vi "PixelFlyTEMP.vi"() -> ()   [LabVIEW 2012]
uses:
  <vilib>/Platform/TimedLoop/XDataNode/timing_clust.ctl
  <vilib>/Platform/TimedLoop/XDataNode/nitl_modes.ctl
  <vilib>/Platform/TimedLoop/XDataNode/wakeup.ctl
  <vilib>/platform/TimedLoop/XDataNode/XDataNode.xnode
  <vilib>/Platform/TimedLoop/XDataNode/XDNodeRunTimeDep.lvlib
panel:
  in  "Tab Control":enum32{"Control", "Advanced"}(tab)
  out "Intensity Graph":dbl[][](graph)
  in  "?":u16(ring) items=["Debug", "Bulb Trigger", "Free Run"]
  in  "bUseBuffer0":bool
  in  "Open StructureIn":T1={"Size"=88, "InterfaceType"=0, "Camera Number"=0, "CameraNumAtInterface"=0, "OpenFlags"=[], "OpenDWFlags"=[], "OpenPtrs"=[]}
  in  "bUseBuffer1":bool
  in  "stop":bool
  in  "stop 2":bool
  out "BufNr0":i16
  out "BufNr1":i16
  out "Bits/pixel":u16
  in  "ROIX1":u16=1 min=1
  in  "ROIY1":u16=1 min=1
  in  "ROIY0":u16=1 min=1
  in  "ROIX0":u16=1 min=1
  in  "DelayTimeBase":u16(ring)=2 items=["nanoseconds", "microseconds", "milliseconds"]
  in  "ExposureTimeBase":u16(ring)=1 items=["nanoseconds", "microseconds", "milliseconds"]
  in  "Exposure":u32=60
  in  "InterfaceType":u16(ring)=6 items=["IEEE1394 - Firewire", "IEEE1394/Firewire", "Matrox Helios Camera Link", "Silicon Software ME3 Camera Link", "National Instruments Camera Link", "Gigabit Ethernet", "USB", "Reserved", "Reserved", "Reserved", "Generic Camera Link with CLSER.DLL"]
  in  "Rate":i32
  in  "StorageMode":bool
  in  "TriggerMode":u16(ring)=2 items=["Auto", "Software", "External sequence start ", "External exposure control"]
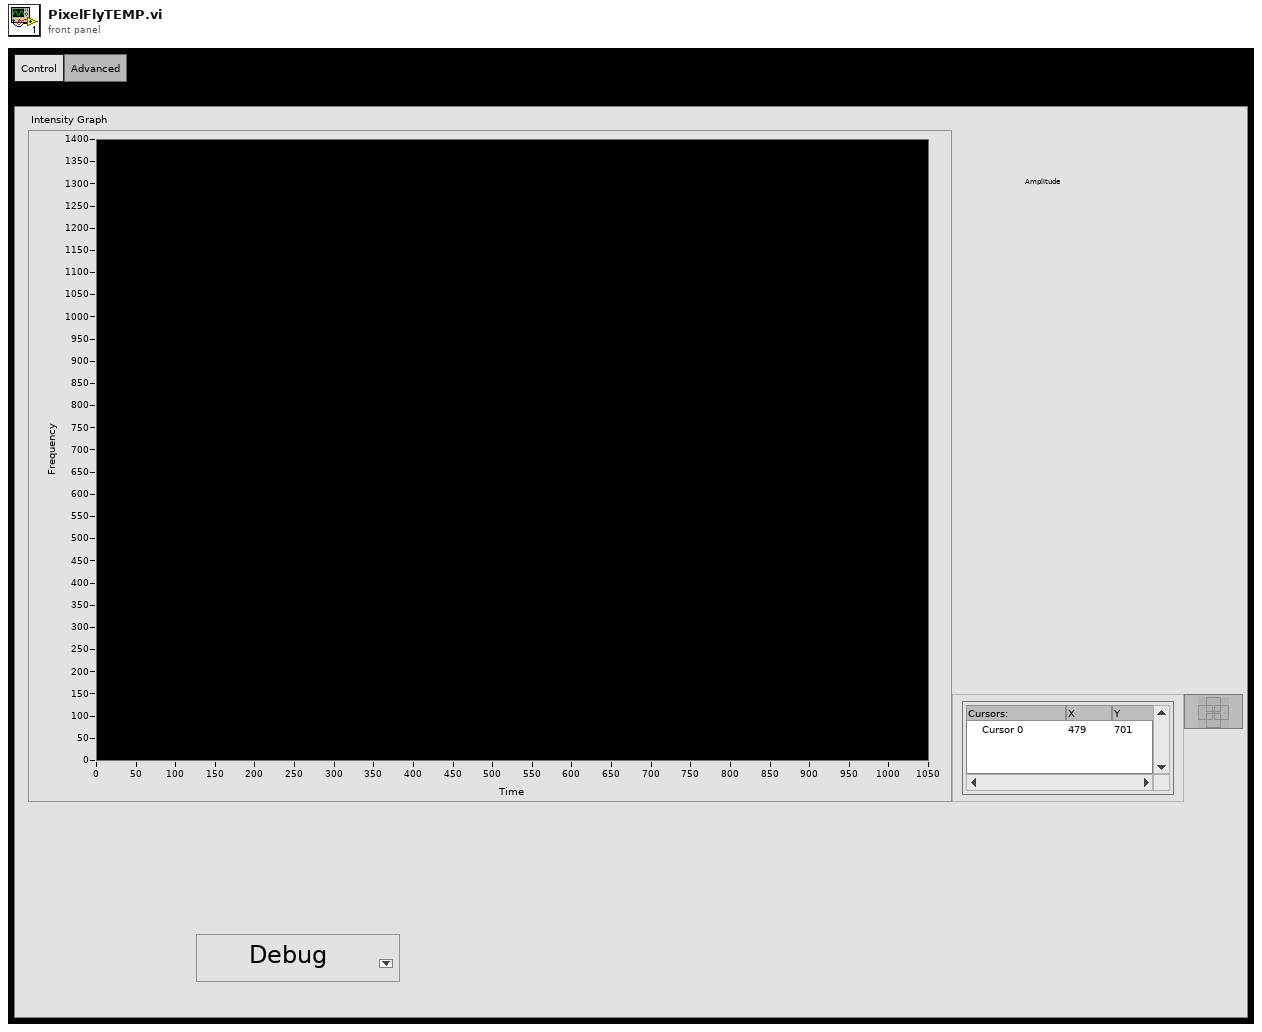
[diagram p1: front panel]
types:
  T1 = cluster{"Size":u16, "InterfaceType":u16, "Camera Number":u16, "CameraNumAtInterface":u16, "OpenFlags":u16[], "OpenDWFlags":u32[], "OpenPtrs":u32[]}
  T2 = typedef "XDNodeRunTimeDep.lvlib/timing_clust.ctl" = cluster{"Expected End [f-1]":u64, "Actual End [f-1]":u64, "Finished Late? [f-1]":bool, "Expected End [i-1]":u64, "Actual End [i-1]":u64, "Finished Late? [i-1]":bool, "Expected Start [i]":u64, "Actual Start [i]":u64, "Expected Start [f]":u64, "Actual Start [f]":u64, "Source Name":string, "Structure Name":string, "Period":i64, "Deadline":i64, "Offset":i64, "Start":i64, "Priority":i32, "Timeout":i32, "Mode":T3, "Wakeup Reason":T4, "Error":errorcluster, "Source Type":string, "Secondary Source Type":string, "Global End Time":u64, "Global Start Time":u64, "Frame Duration":u64, "Iteration Duration":u64, "Assigned CPU":i32, "I/O Scan Engine Mode":u32}
  T3 = typedef "XDNodeRunTimeDep.lvlib/nitl_modes.ctl" = enum32{"No Change", "Process missed periods, maintain original phase", "Discard missed periods, maintain original phase", "Process missed periods, ignore original phase", "Discard missed periods, ignore original phase"}
  T4 = typedef "XDNodeRunTimeDep.lvlib/wakeup.ctl" = enum32{"Normal", "Aborted", "Asynchronous wakeup", "Timing source error", "Timed loop error", "Timeout"}
  T5 = cluster{"Size":u16, "CamType":u16, "CamSubType":u16, "SerialNumber":u32, "HWVersion":u32, "FWVersion":u32, "InterfaceType":u16, "HardwareVersion":cluster{"BoardNum":u16, "HWVersions":cluster{"BoardName":string, "BatchNumber":u16, "MinorRevision":u8, "MajorRevision":u8, "Variant":u16}[]}, "FirmwareVersion":cluster{"DeviceNum":u16, "FWVersions":cluster{"DeviceName":string, "MinorRevision":u8, "MajorRevision":u8, "Variant":u16}[]}}
  T6 = cluster{"Size":u16, "SensorTypeDESC":u16, "SensorSubtypeDESC":u16, "MaxHorizontalResStdDESC":u16, "MaxVerticalResStdDESC":u16, "MaxHorizontalResExtDESC":u16, "MaxVerticalResExtDESC":u16, "DynResDESC":u16, "MaxBinHorzDESC":u16, "BinHorzStepDESC":bool, "MaxBinVertDESC":u16, "BinVertStepDESC":bool, "ROIHorzStepDESC":u16, "ROIVertStepDESC":u16, "NumADCDESC":u16, "IRDESC":bool, "MinDelayDESC":u32, "MaxDelayDESC":u32, "MinDelayStepDESC":u32, "MinExpoDESC":u32, "MaxExpoDESC":u32, "MinExpoStepDESC":u32, "MinDelayIRDESC":u32, "MaxDelayIRDESC":u32, "MinExpoIRDESC":u32, "MaxExpoIRDESC":u32, "TimeTableDESC":bool, "DoubleImageDESC":bool, "MinCoolSetDESC":i16, "MaxCoolSetDESC":i16, "MDefaultCoolSetDESC":i16, "PowerDownModeDESC":bool, "OffsetRegDESC":bool, "ColorPattern":cluster{"UpperLeftColor":u8, "UpperRightColor":u8, "LowerLeftColor":u8, "LowerRightColor":u8}, "PatternTypeDESC":bool, "PixelRates":u32[], "CoversionFactors":u16[], "Reserved":u32[], "NoiseFilterCapable":bool, "HotPixelCapable":bool, "HotPixelWithNoiseFilter":bool, "ASCIITimeCapable":bool, "Extended Description":bool, "Get Extended":bool, "Reserved Flag 1":bool, "Reserved Flag 2":bool}
  T7 = cluster{u16[][], "XResAct":u16, "YResAct":u16, "BufNrOut":i16, "BufNrOut":i16, "ErrorOut":errorcluster, "hout":u64, "Bits/pixel":u16}
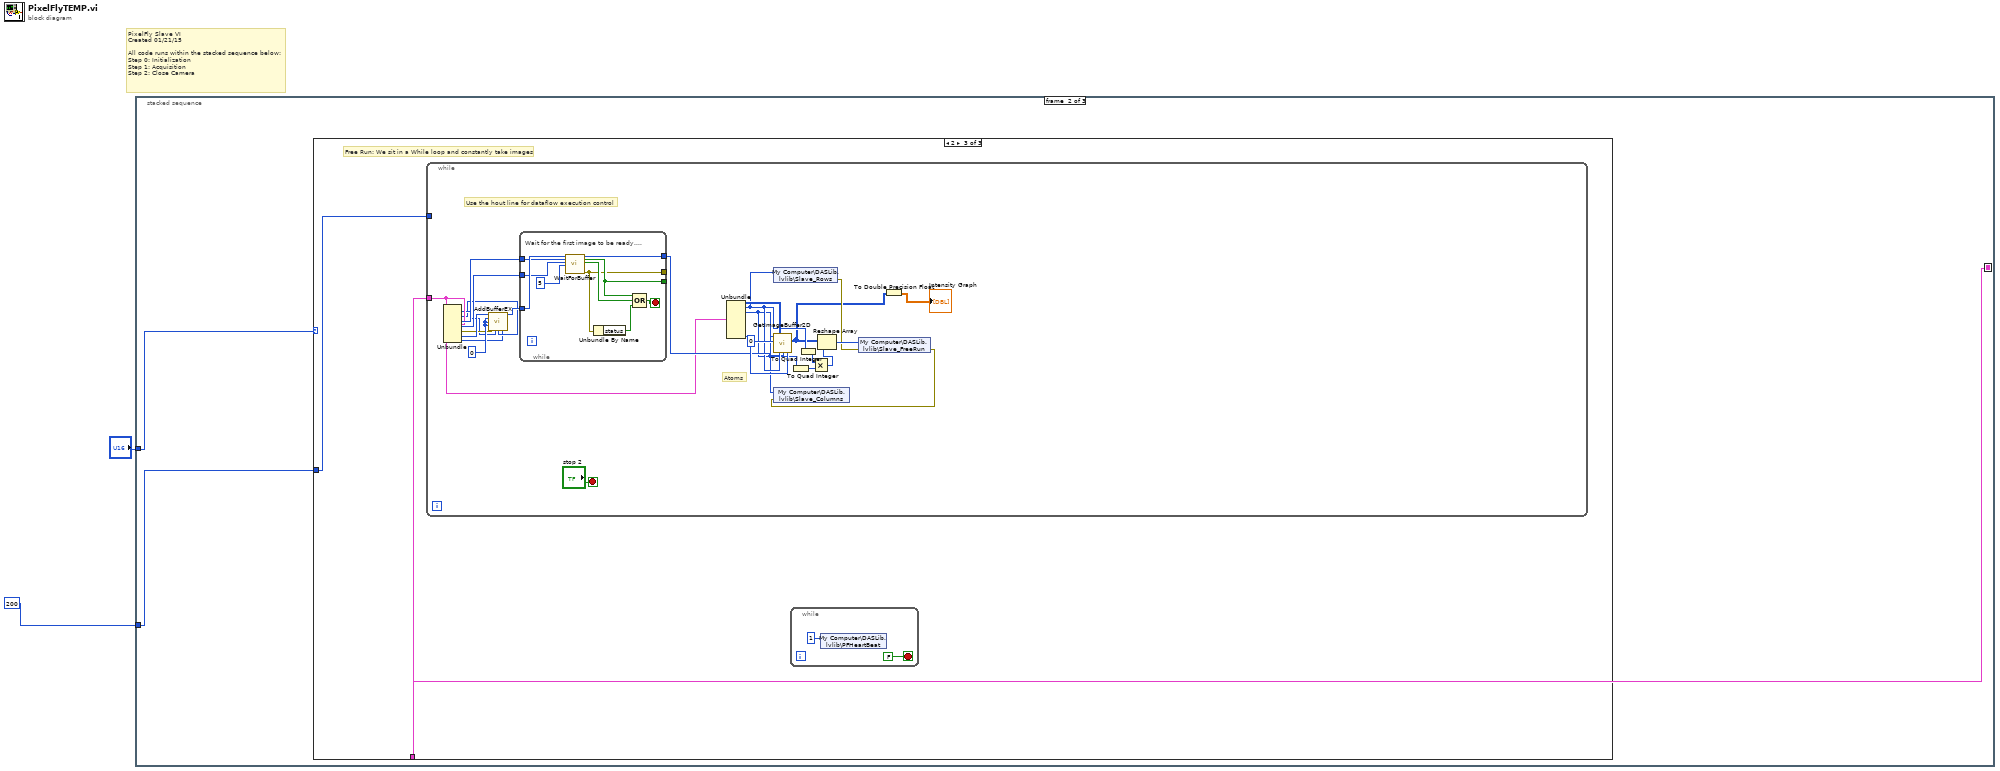
[diagram p0: block diagram]
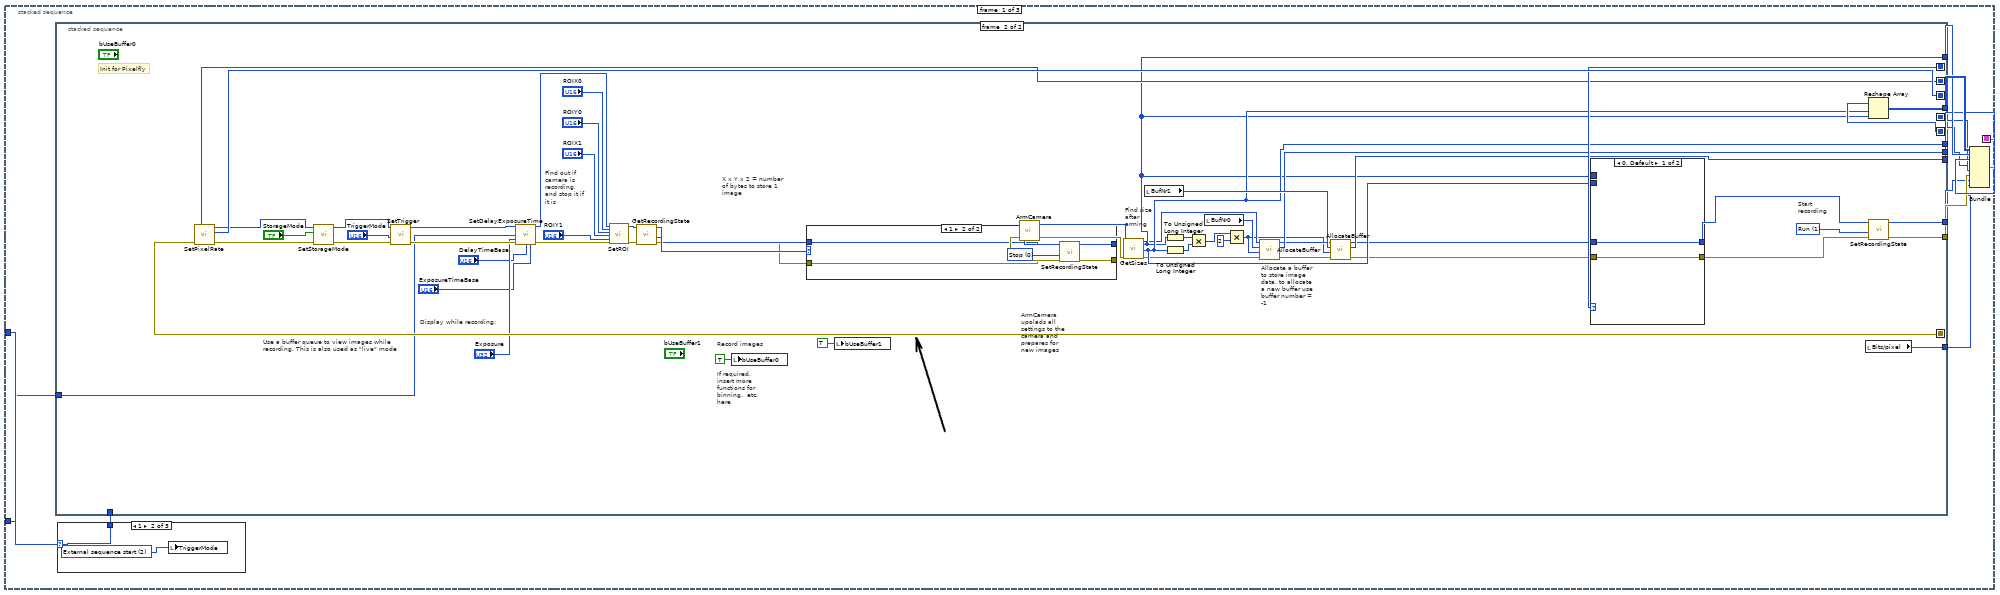
[diagram p2: hidden frame]
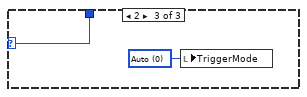
[diagram p4: hidden frame]
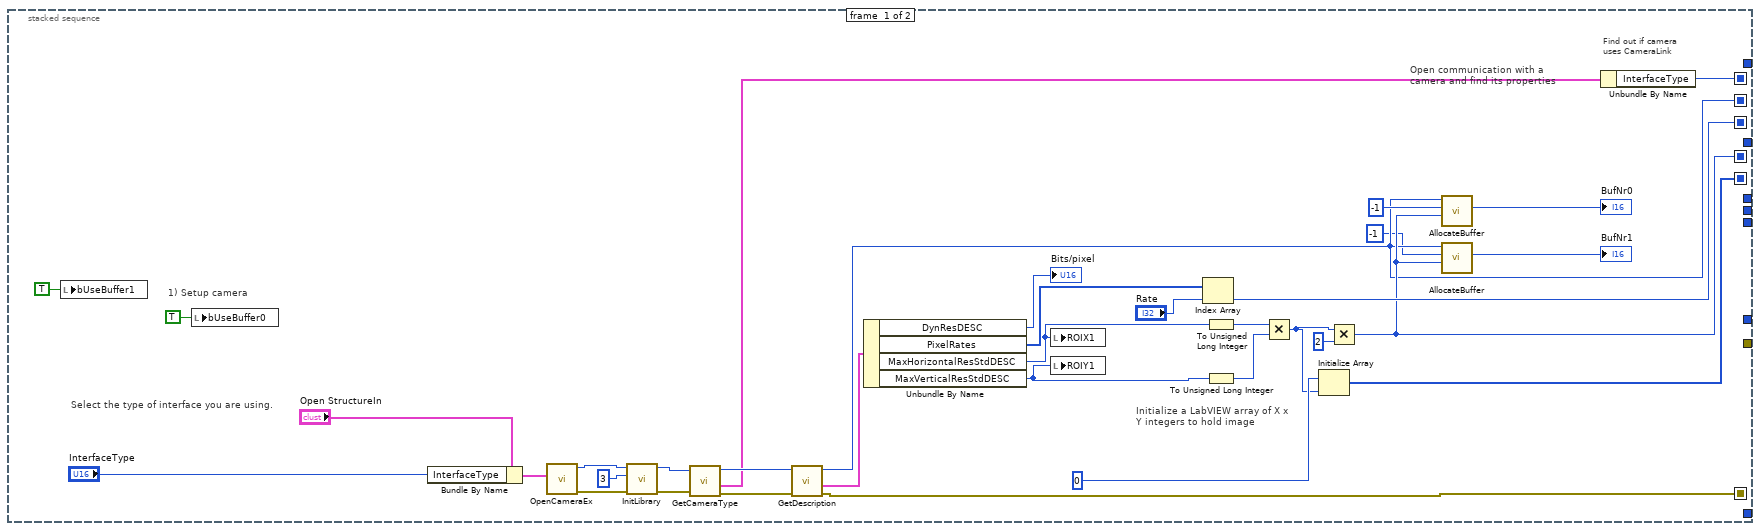
[diagram p5: hidden frame]
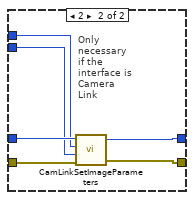
[diagram p6: hidden frame]
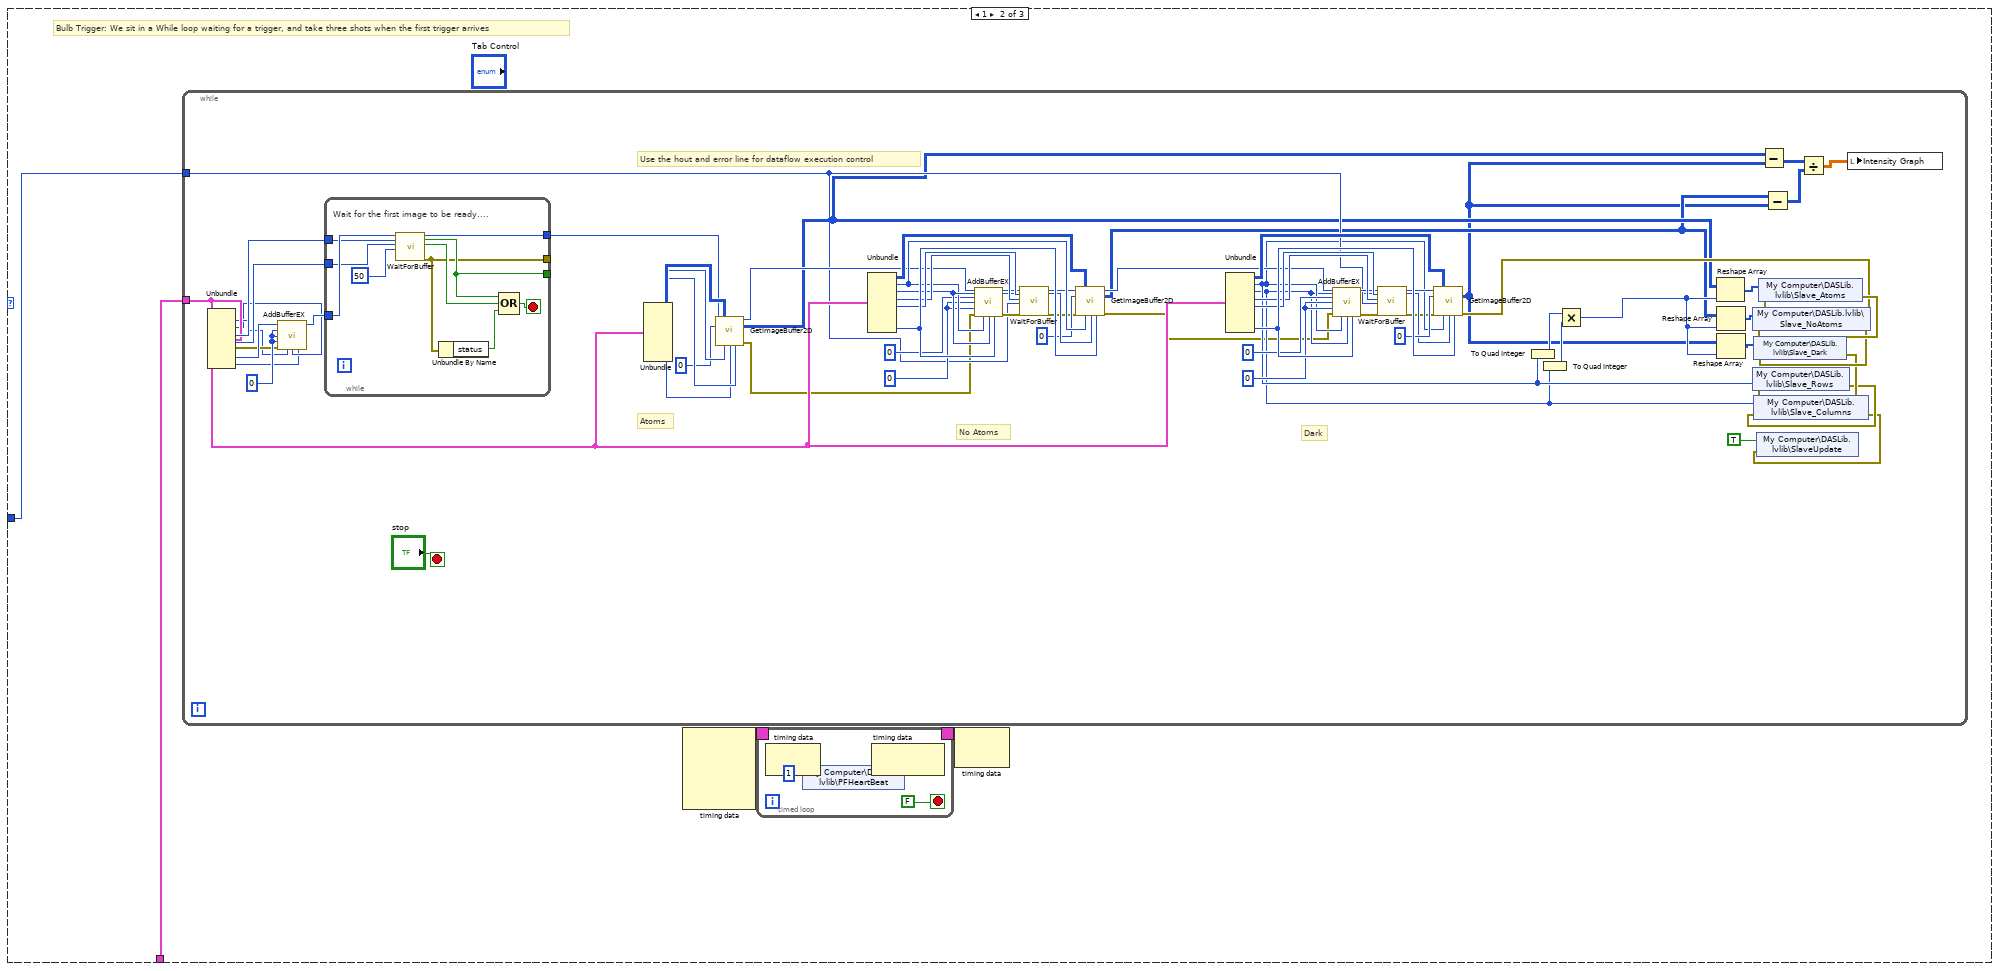
[diagram p9: hidden frame]
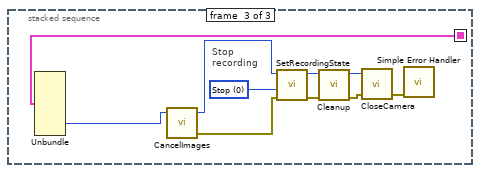
[diagram p10: hidden frame]
diagram:
  # "PixelFly Slave VI\nCreated 01/21/15\n\nAll code runs within the stacked sequence below:\nStep 0: Initialization\nStep 1: Acquisition\nStep 2: Close Camera"
  n1 = stacked-sequence {
    seq-local: [w6 _ _] -> [_ w128 w257]
    tunnel: "?" -> [w5 w129 _]
    tunnel: 200 -> [w3 w127 _]
    frame #0 {
      n2 = case shown="1" w5 {
        selector: w5 -> [w15 w16 w18]
        tunnel: [w15 w16 w18] -> w4
        frame 0, Default {
        }
        frame 1 {
          w17 = u16 2 items=["Auto", "Software", "External sequence start ", "External exposure control"] ("TriggerMode")
          n3 = local write "TriggerMode"(w17) -> ()
        }
        frame 2 {
          w19 = u16 0 items=["Auto", "Software", "External sequence start ", "External exposure control"] ("TriggerMode")
          n4 = local write "TriggerMode"(w19) -> ()
        }
      }
      n5 = stacked-sequence {
        seq-local: [w50 _] -> [_ w108]
        seq-local: [w31 _] -> [_ _]
        seq-local: [w43 _] -> [_ w110]
        seq-local: [w30 _] -> [_ w105]
        seq-local: [w42 _] -> [_ w111]
        seq-local: [w41 _] -> [_ w109]
        tunnel: [_ w104] -> w14
        tunnel: [_ w100] -> w13
        tunnel: [_ w103] -> w12
        tunnel: [_ w102] -> w11
        tunnel: [_ w101] -> w10
        tunnel: [_ w99] -> w8
        tunnel: [_ w98] -> w9
        tunnel: [_ w97] -> w7
        tunnel: w4 -> [_ _]
        tunnel: w3 -> [_ w54]
        frame #0 {
          # "Select the type of interface you are using."
          # "1) Setup camera"
          # "Find out if camera uses CameraLink"
          # "Initialize a LabVIEW array of X x Y integers to hold image"
          # "Open communication with a camera and find its properties"
          n6 = local write "bUseBuffer1"(TRUE) -> ()
          n7 = local write "bUseBuffer0"(TRUE) -> ()
          n8 = Bundle By Name(cluster="Open StructureIn", "InterfaceType"="InterfaceType") -> (w38:T1)
          n9 = call "OpenCameraEx.vi"("OpenStructureIn"=w38) -> ("error out"=w22:errorcluster, "hout"=w23:u64)  [unwired: 3 in, 2 out]
          n10 = call "InitLibrary.vi"("error in (no error)"=w22, "InterfaceType"=u32 3, "ph"=w23) -> ("error out"=w20:errorcluster, "hout"=w21:u64)  [unwired: 7 in]
          n11 = call "GetCameraType.vi"("ph"=w21, "error in (no error)"=w20) -> ("hout"=w47:u64, "CameraType"=w45:T5, "error out"=w46:errorcluster)  [unwired: 1 in, 1 out]
          n12 = call "GetDescription.vi"("ErrorIn"=w46, "ph"=w47) -> ("ErrorOut"=w42:errorcluster, "Description"=w49:T6, "hout"=w30:u64)  [unwired: 2 in, 1 out]
          n13 = Unbundle By Name(w49) -> ("DynResDESC"=→"Bits/pixel":u16, "PixelRates"=w44:u32[], "MaxHorizontalResStdDESC"=w36:u16, "MaxVerticalResStdDESC"=w35:u16)
          n14 = local write "ROIX1"(w36) -> ()
          n15 = local write "ROIY1"(w35) -> ()
          n16 = Index Array(array=w44, index="Rate") -> (element=w43:u32)
          n17 = To Unsigned Long Integer(number=w36) -> (unsigned 32bit integer=w33:u32)
          n18 = To Unsigned Long Integer(number=w35) -> (unsigned 32bit integer=w32:u32)
          n19 = Multiply(x=w33, y=w32) -> (x*y=w51:u32)
          n20 = Initialize Array(u16 0 ("Element Data"), w51) -> (w50:u16[])
          n21 = Multiply(x=w51, y=u32 2) -> (x*y=w31:u32)
          n22 = call "AllocateBuffer.vi"("Size"=w31, "BufNr"=i16 -1, "ph"=w30) -> ("BufNrOut"=→"BufNr0":i16)  [unwired: 3 in, 5 out]
          n23 = call "AllocateBuffer.vi"("Size"=w31, "BufNr"=-1, "ph"=w30) -> ("BufNrOut"=→"BufNr1":i16)  [unwired: 3 in, 5 out]
          n24 = Unbundle By Name(w45) -> ("InterfaceType"=w41:u16)
        }
        frame #1 {
          w96 = u16 1 items=["Stop", "Run"] ("RecordingState")
          # "Init for Pixelfly"
          # "Record images"
          # "Start recording"
          # "Allocate a buffer to store image data. to allocate a new buffer use buffer number = -1"
          # "Find size after arming"
          # "ArmCamera upolads all settings to the camera and prepares for new images"
          # "Find out if camera is recording, and stop it if it is"
          # "If required, insert more functions for binning.  etc. here"
          # "X x Y x 2 = number of bytes to store 1 image"
          # "Use a buffer queue to view images while recording. This is also used as \"live\" mode"
          # "Display while recording:"
          n25 = call "SetPixelRate.vi"("error in (no error)"=w111, "PixelRate"=w110, "ph"=w105) -> ("error out"=w94:errorcluster, "hout"=w95:u64)  [unwired: 2 in, 1 out]
          n26 = call "SetStorageMode.vi"("error in (no error)"=w94, "StorageMode"="StorageMode", "ph"=w95) -> ("error out"=w86:errorcluster, "hout"=w87:u64)  [unwired: 2 in, 1 out]
          n27 = call "SetTrigger.vi"("error in (no error)"=w86, "TriggerMode"="TriggerMode", "ph"=w87) -> ("error out"=w79:errorcluster, "hout"=w80:u64)  [unwired: 2 in, 1 out]
          n28 = call "SetDelayExposureTime.vi"("ph"=w80, "Delay"=w54, "Exposure"="Exposure", "error in (no error)"=w79, "DelayTimeBase"="DelayTimeBase", "ExposureTimeBase"="ExposureTimeBase") -> ("hout"=w69:u64, "error out"=w67:errorcluster)  [unwired: 7 in, 1 out]
          n29 = call "SetROI.vi"("ph"=w69, "ROIX0"="ROIX0", "ROIY0"="ROIY0", "ROIX1"="ROIX1", "ROIY1"="ROIY1", "error in (no error)"=w67) -> ("hout"=w68:u64, "error out"=w66:errorcluster)  [unwired: 12 in]
          n30 = call "GetRecordingState.vi"("ErrorIn"=w66, "ph"=w68) -> ("ErrorOut"=w90:errorcluster, "RecordingState"=w92:u16, "hout"=w91:u64)  [unwired: 2 in, 1 out]
          n31 = local write "bUseBuffer0"(TRUE) -> ()
          n32 = case shown="1" w92 {
            tunnel: w91 -> [w121 w125]
            tunnel: w90 -> [w120 w124]
            tunnel: [w121 w123] -> w89
            tunnel: [w120 w122] -> w88
            frame 0, Default {
            }
            frame 1 {
              w126 = u16 0 items=["Stop", "Run"] ("RecordingState")
              n33 = call "SetRecordingState.vi"("ErrorIn"=w124, "RecordingState"=w126, "ph"=w125) -> ("ErrorOut"=w122:errorcluster, "hout"=w123:u64)  [unwired: 2 in, 1 out]
            }
          }
          n34 = local write "bUseBuffer1"(TRUE) -> ()
          n35 = call "ArmCamera.vi"("error in (no error)"=w88, "ph"=w89) -> ("error out"=w84:errorcluster, "hout"=w85:u64)  [unwired: 1 in, 1 out]
          n36 = call "GetSizes.vi"("ph"=w85, "ErrorIn"=w84) -> ("hout"=w81:u64, "XResAct"=w100:u16, "YResAct"=w103:u16, "ErrorOut"=w83:errorcluster)  [unwired: 11 in, 3 out]
          n37 = local read "BufNr1"() -> (w107:i16)
          n38 = To Unsigned Long Integer(number=w100) -> (unsigned 32bit integer=w70:u32)
          n39 = To Unsigned Long Integer(number=w103) -> (unsigned 32bit integer=w71:u32)
          n40 = Multiply(x=w70, y=w71) -> (x*y=w72:u32)
          n41 = local read "BufNr0"() -> (w106:i16)
          n42 = Multiply(x=w72, y=u32 2) -> (x*y=w57:u32)
          n43 = call "AllocateBuffer.vi"("error in (no error)"=w83, "Size"=w57, "BufNr"=w106, "ph"=w81) -> ("error out"=w61:errorcluster, "BufNrOut"=w102:i16, "hout"=w59:u64)  [unwired: 2 in, 3 out]
          n44 = call "AllocateBuffer.vi"("error in (no error)"=w61, "Size"=w57, "BufNr"=w107, "ph"=w59) -> ("error out"=w60:errorcluster, "BufNrOut"=w101:i16, "hout"=w58:u64)  [unwired: 2 in, 3 out]
          n45 = case shown="0, Default" w109 {
            tunnel: w60 -> [w112 w119]
            tunnel: [w112 w118] -> w75
            tunnel: w58 -> [w113 w117]
            tunnel: [w113 w116] -> w74
            tunnel: w103 -> [_ w115]
            tunnel: w100 -> [_ w114]
            frame 0, Default {
            }
            frame 2 {
              # "Only necessary if the interface is Camera Link"
              n46 = call "CamLinkSetImageParameters.vi"("error in (no error)"=w119, "YRes"=w115, "XRes"=w114, "ph"=w117) -> ("error out"=w118:errorcluster, "hout"=w116:u64)  [unwired: 1 out]
            }
          }
          n47 = local read "Bits/pixel"() -> (w97:u16)
          n48 = Reshape Array(w108, w103, w100) -> (w104:u16[][])
          n49 = call "SetRecordingState.vi"("ErrorIn"=w75, "RecordingState"=w96, "ph"=w74) -> ("ErrorOut"=w98:errorcluster, "hout"=w99:u64)  [unwired: 2 in, 1 out]
        }
      }
      n50 = Bundle(w14, "XResAct"=w13, "YResAct"=w12, "BufNrOut"=w10, "BufNrOut"=w11, "ErrorOut"=w9, "hout"=w8, "Bits/pixel"=w7) -> (w6:T7)  [unwired: 1 in]
    }
    frame #1 {
      n51 = case shown="2" w129 {
        tunnel: w128 -> [_ w133 w218]
        tunnel: w127 -> [_ w132 w217]
        frame 0, Default {
          # "Debug Mode: Do nothing here\nProceeds directly to closing the camera"
        }
        frame 1 {
          # "Bulb Trigger: We sit in a While loop waiting for a trigger, and take three shots when the first trigger arrives"
          n52 = while {
            tunnel: w133 -> [w169]
            tunnel: w132 -> [w168]
            stop <- "stop" stop-if-true
            w174 = 0
            w185 = 0
            w201 = 0
            # "Dark"
            # "No Atoms"
            # "Atoms"
            # "Use the hout and error line for dataflow execution control"
            n53 = Unbundle(w169) -> ("XResAct"=w167:u16, "YResAct"=w166:u16, "BufNrOut"=w197:i16, "BufNrOut"=w196:i16, "ErrorOut"=w199:errorcluster, "hout"=w200:u64, "Bits/pixel"=w165:u16)  [unwired: 1 out]
            n54 = call "AddBufferEX.vi"("ph"=w200, "BuffNr"=w201, "1stImage"=w201, "LastImage"=w201, "error in (no error)"=w199, "XRes"=w167, "YRes"=w166, "BitPerPixel"=w165) -> ("hout"=w198:u64)  [unwired: 5 in, 2 out]
            n55 = while {
              tunnel: [w212] -> _
              tunnel: [w215] -> _
              tunnel: w198 -> [w210]
              tunnel: w197 -> [w209]
              tunnel: w196 -> [w208]
              tunnel: [w207] -> w195
              stop <- w216 stop-if-true
              # "Wait for the first image to be ready...."
              n56 = call "WaitForBuffer.vi"("ph"=w210, "sBufNr"=w209, "sBufNr 2"=w208, "timeout"=50) -> ("hout"=w207:u64, "Buffer_Ready"=w215:bool, "Buffer_Ready 2"=w214:bool, "error out"=w212:errorcluster)  [unwired: 11 in, 1 out]
              n57 = Unbundle By Name(w212) -> ("status"=w211:bool)
              n58 = Compound Arithmetic op=OR(w215, w214, w211) -> (w216:bool)
            }
            n59 = Unbundle(w169) -> (w206:u16[][], "XResAct"=w204:u16, "YResAct"=w194:u16, "Bits/pixel"=w205:u16)  [unwired: 4 out]
            n60 = call "GetImageBuffer2D.vi"("ph"=w195, "BuffIn"=w206, "BuffNr"=i16 0, "xRes"=w204, "yRes"=w194, "Bitresolution"=w205) -> ("hout"=w181:u64, "BuffOut"=w145:u16[][], "error out"=w157:errorcluster)  [unwired: 6 in, 1 out]
            n61 = Unbundle(w169) -> (w193:u16[][], "XResAct"=w188:u16, "YResAct"=w189:u16, "BufNrOut"=w190:i16, "BufNrOut"=w191:i16, "Bits/pixel"=w192:u16)  [unwired: 2 out]
            n62 = call "AddBufferEX.vi"("ph"=w181, "BuffNr"=i16 0, "1stImage"=w185, "LastImage"=w185, "error in (no error)"=w157, "XRes"=w188, "YRes"=w189, "BitPerPixel"=w192) -> ("hout"=w183:u64, "error out"=w184:errorcluster)  [unwired: 5 in, 1 out]
            n63 = call "WaitForBuffer.vi"("ph"=w183, "sBufNr"=w191, "sBufNr 2"=w190, "timeout"=w168, "error in (no error)"=w184) -> ("hout"=w182:u64, "error out"=w158:errorcluster)  [unwired: 10 in, 3 out]
            n64 = call "GetImageBuffer2D.vi"("ph"=w182, "BuffIn"=w193, "BuffNr"=i16 0, "error in (no error)"=w158, "xRes"=w188, "yRes"=w189, "Bitresolution"=w192) -> ("hout"=w170:u64, "BuffOut"=w144:u16[][], "error out"=w156:errorcluster)  [unwired: 5 in, 1 out]
            n65 = Unbundle(w169) -> (w180:u16[][], "XResAct"=w164:u16, "YResAct"=w163:u16, "BufNrOut"=w177:i16, "BufNrOut"=w178:i16, "Bits/pixel"=w179:u16)  [unwired: 2 out]
            n66 = call "AddBufferEX.vi"("ph"=w170, "BuffNr"=i16 0, "1stImage"=w174, "LastImage"=w174, "error in (no error)"=w156, "XRes"=w164, "YRes"=w163, "BitPerPixel"=w179) -> ("hout"=w172:u64, "error out"=w173:errorcluster)  [unwired: 5 in, 1 out]
            n67 = call "WaitForBuffer.vi"("ph"=w172, "sBufNr"=w178, "sBufNr 2"=w177, "timeout"=w168, "error in (no error)"=w173) -> ("hout"=w171:u64, "error out"=w155:errorcluster)  [unwired: 10 in, 3 out]
            n68 = call "GetImageBuffer2D.vi"("ph"=w171, "BuffIn"=w180, "BuffNr"=i16 0, "error in (no error)"=w155, "xRes"=w164, "yRes"=w163, "Bitresolution"=w179) -> ("BuffOut"=w143:u16[][], "error out"=w153:errorcluster)  [unwired: 5 in, 2 out]
            n69 = To Quad Integer(1:w164) -> (0:w146:i64)
            n70 = To Quad Integer(1:w163) -> (0:w147:i64)
            n71 = Multiply(x=w146, y=w147) -> (x*y=w162:i64)
            n72 = Reshape Array(w145, w162) -> (w161:u16[])
            n73 = Reshape Array(w144, w162) -> (w160:u16[])
            n74 = Reshape Array(w143, w162) -> (w159:u16[])
            n75 = shared-variable "My Computer\\DASLib.lvlib\\Slave_Atoms"(w161, error in=w153) -> (error out=w154:errorcluster)
            n76 = shared-variable "My Computer\\DASLib.lvlib\\Slave_NoAtoms"(w160, error in=w154) -> (error out=w152:errorcluster)
            n77 = shared-variable "My Computer\\DASLib.lvlib\\Slave_Dark"(w159, error in=w152) -> (error out=w151:errorcluster)
            n78 = shared-variable "My Computer\\DASLib.lvlib\\Slave_Rows"(w164, error in=w151) -> (error out=w150:errorcluster)
            n79 = shared-variable "My Computer\\DASLib.lvlib\\Slave_Columns"(w163, error in=w150) -> (error out=w148:errorcluster)
            n80 = shared-variable "My Computer\\DASLib.lvlib\\SlaveUpdate"(TRUE ("SlaveUpdate"), error in=w148) -> ()  [unwired: 1 out]
            n81 = Subtract(x=w145, y=w143) -> (x-y=w141:u16[][])
            n82 = Subtract(x=w144, y=w143) -> (x-y=w142:u16[][])
            n83 = Divide(x=w141, y=w142) -> (x/y=w140:dbl[][])
            n84 = local write "Intensity Graph"(w140) -> ()
          }
          n85 = node-c288() -> (w131:T2)  [unwired: 4 in]
          n86 = timed-loop {
            timing: w131 -> [_]
            timing-out: [_] -> w130
            stop <- FALSE stop-if-true
            n87 = node-c288() -> ()  [unwired: 1 in, 1 out]
            n88 = shared-variable "My Computer\\DASLib.lvlib\\PFHeartBeat"(i16 1 ("PFHeartBeat")) -> ()  [unwired: 1 in, 1 out]
            n89 = node-c288() -> ()  [unwired: 1 in, 1 out]
          }
          n90 = node-c288(w130) -> ()  [unwired: 1 out]
        }
        frame 2 {
          # "Free Run: We sit in a While loop and constantly take images"
          n91 = while {
            tunnel: w218 -> [w234]
            tunnel: w217 -> [_]
            stop <- "stop 2" stop-if-true
            w241 = 0
            # "Atoms"
            # "Use the hout line for dataflow execution control"
            n92 = Unbundle(w234) -> ("XResAct"=w233:u16, "YResAct"=w232:u16, "BufNrOut"=w237:i16, "BufNrOut"=w236:i16, "ErrorOut"=w239:errorcluster, "hout"=w240:u64, "Bits/pixel"=w231:u16)  [unwired: 1 out]
            n93 = call "AddBufferEX.vi"("ph"=w240, "BuffNr"=w241, "1stImage"=w241, "LastImage"=w241, "error in (no error)"=w239, "XRes"=w233, "YRes"=w232, "BitPerPixel"=w231) -> ("hout"=w238:u64)  [unwired: 5 in, 2 out]
            n94 = while {
              tunnel: [w251] -> _
              tunnel: [w254] -> _
              tunnel: w238 -> [w249]
              tunnel: w237 -> [w248]
              tunnel: w236 -> [w247]
              tunnel: [w246] -> w235
              stop <- w255 stop-if-true
              # "Wait for the first image to be ready...."
              n95 = call "WaitForBuffer.vi"("ph"=w249, "sBufNr"=w248, "sBufNr 2"=w247, "timeout"=5) -> ("hout"=w246:u64, "Buffer_Ready"=w254:bool, "Buffer_Ready 2"=w253:bool, "error out"=w251:errorcluster)  [unwired: 11 in, 1 out]
              n96 = Unbundle By Name(w251) -> ("status"=w250:bool)
              n97 = Compound Arithmetic op=OR(w254, w253, w250) -> (w255:bool)
            }
            n98 = Unbundle(w234) -> (w245:u16[][], "XResAct"=w229:u16, "YResAct"=w228:u16, "Bits/pixel"=w244:u16)  [unwired: 4 out]
            n99 = call "GetImageBuffer2D.vi"("ph"=w235, "BuffIn"=w245, "BuffNr"=i16 0, "xRes"=w229, "yRes"=w228, "Bitresolution"=w244) -> ("BuffOut"=w222:u16[][])  [unwired: 6 in, 3 out]
            n100 = shared-variable "My Computer\\DASLib.lvlib\\Slave_Rows"(w229) -> (error out=w226:errorcluster)  [unwired: 1 in]
            n101 = To Quad Integer(1:w228) -> (0:w223:i64)
            n102 = To Quad Integer(1:w229) -> (0:w224:i64)
            n103 = Multiply(x=w224, y=w223) -> (x*y=w230:i64)
            n104 = Reshape Array(w222, w230) -> (w227:u16[])
            n105 = shared-variable "My Computer\\DASLib.lvlib\\Slave_FreeRun"(w227, error in=w226) -> (error out=w225:errorcluster)
            n106 = shared-variable "My Computer\\DASLib.lvlib\\Slave_Columns"(w228, error in=w225) -> ()  [unwired: 1 out]
            n107 = To Double Precision Float(number=w222) -> (double precision float=→"Intensity Graph":dbl[][])
          }
          n108 = while {
            stop <- FALSE stop-if-true
            n109 = shared-variable "My Computer\\DASLib.lvlib\\PFHeartBeat"(i16 1 ("PFHeartBeat")) -> ()  [unwired: 1 in, 1 out]
          }
        }
      }
    }
    frame #2 {
      w263 = u16 0 items=["Stop", "Run"] ("RecordingState")
      # "Stop recording"
      n110 = Unbundle(w257) -> ("hout"=w256:u64)  [unwired: 7 out]
      n111 = call "CancelImages.vi"("ph"=w256) -> ("error out"=w265:errorcluster, "hout"=w264:u64)  [unwired: 2 in, 1 out]
      n112 = call "SetRecordingState.vi"("ErrorIn"=w265, "RecordingState"=w263, "ph"=w264) -> ("ErrorOut"=w258:errorcluster, "hout"=w259:u64)  [unwired: 2 in, 1 out]
      n113 = call "Cleanup.vi"("error in (no error)"=w258, "ph"=w259) -> ("error out"=w261:errorcluster, "hout"=w260:u64)  [unwired: 8 in]
      n114 = call "CloseCamera.vi"("ErrorIn"=w261, "Handle in"=w260) -> ("ErrorOut"=w262:errorcluster)  [unwired: 1 in, 2 out]
      n115 = call <vilib>:"Simple Error Handler.vi"("error in (no error)"=w262) -> ()  [unwired: 4 in, 5 out]
    }
  }
